vi "Draw plane.vi"(3 "Number (0)":u8) -> (0 "Modify object":refnum<vi>, 1 "Draw object":refnum<vi>)   [LabVIEW 2017]
uses:
  <vilib>/Utility/miscctls.llb/LVRGBAColorTypeDef.ctl
  <vilib>/picture/3D Picture Control/Object/Create Object (name).vi
  <vilib>/picture/3D Picture Control/NI_3D Picture Control.lvlib
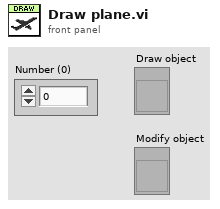
[diagram p1: front panel]
types:
  T1 = cluster{"Red":sgl, "Green":sgl, "Blue":sgl, "Alpha":sgl}
  T2 = enum16{"Overall", "Per Primitive", "Per Vertex", "Binding Off"}
  T3 = typedef "LVRGBAColorTypeDef.ctl" = cluster{"Red":sgl, "Green":sgl, "Blue":sgl, "Alpha":sgl}
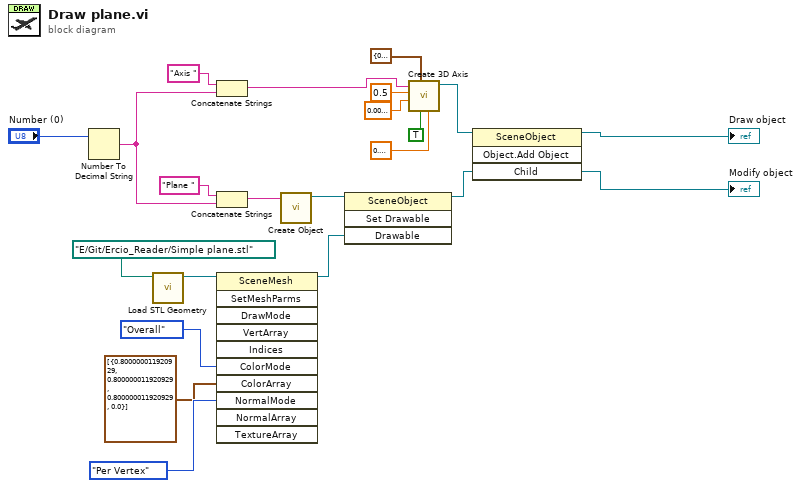
[diagram p0: block diagram]
diagram:
  n1 = Number To Decimal String(number="Number (0)") -> (decimal integer string=w3:string)  [unwired: 1 in]
  n2 = call <vilib>:"Load STL Geometry.vi"("Model File"=path "E:/Git/Ercio_Reader/Simple plane.stl" ("Path Control")) -> ("New Mesh Refnum"=w14:refnum<vi>)  [unwired: 9 in, 1 out]
  n3 = Concatenate Strings("Axis ", w3) -> (w2:string)
  n4 = Concatenate Strings("Plane " ("Name"), w3) -> (w1:string)
  n5 = invoke class="SceneMesh" method="SetMeshParms"(reference=w14, "ColorMode"=T2."Overall" ("Color Binding Mode"), "ColorArray"=T3[] [{"Red"=0.8, "Green"=0.8, "Blue"=0.8, "Alpha"=0.0}] ("Color Array"), "NormalMode"=T2."Per Vertex" ("Normal Binding Mode")) -> (reference out=w15:refnum<vi>)  [unwired: 7 in, 10 out]
  n6 = call-poly <vilib>:"Create Object.vi"("Name"=w1) -> ("Scene:New Object"=w8:refnum<vi>)  [unwired: 9 in, 1 out]
  n7 = invoke class="SceneObject" method="Set Drawable"(reference=w8, "Drawable"=w15) -> (reference out=w20:refnum<vi>)  [unwired: 2 in, 3 out]
  n8 = call <vilib>:"Create 3D Axis.vi"("Character Size"=sgl 0.2, "Axis label?"=TRUE, "Color"=T1 {"Red"=0.4, "Green"=0.4, "Blue"=0.4, "Alpha"=1.0}, "Radius"=sgl 0.01, "Length"=sgl 0.5, "Name"=w2) -> ("New Object Refnum"=w10:refnum<vi>)  [unwired: 4 in, 1 out]
  n9 = invoke class="SceneObject" method="Object.Add Object"(reference=w10, "Child"=w20) -> (reference out=→"Draw object":refnum<vi>, "Child"=→"Modify object":refnum<vi>)  [unwired: 2 in, 2 out]
